vi "test Accessors.vi"(8 "error in (no error)":errorcluster, 11 "TestCase in":refnum<class "Buffers Tests.lvclass">) -> (0 "error out":errorcluster, 3 "TestCase out":refnum<class "Buffers Tests.lvclass">)   [LabVIEW 2017, in "Buffers Tests.lvclass"]
uses:
  Buffers Tests.lvclass
  Buffers Tests.lvclass/Buffers Tests.ctl
  Classes/Buffers/Buffers.lvclass/Buffers.ctl
  Classes/Buffer/Buffer.lvclass
  C:/Git/DSF/LabVIEW-Memory/Source/Classes/Pointer/Pointer.lvclass
  LabVIEW-Memory/Source/Classes/Pointer/Get Address.vi
  LabVIEW-Memory/Source/Classes/Pointer/Get Size.vi
  <vilib>/addons/_JKI Toolkits/VI Tester/TestCase.llb/TestCase.lvclass
  Classes/Buffers/Buffers.lvclass
  C:/Program Files (x86)/National Instruments/LabVIEW 2017/vi.lib/addons/_JKI Toolkits/VI Tester/TestCase.llb/TestCase.lvclass
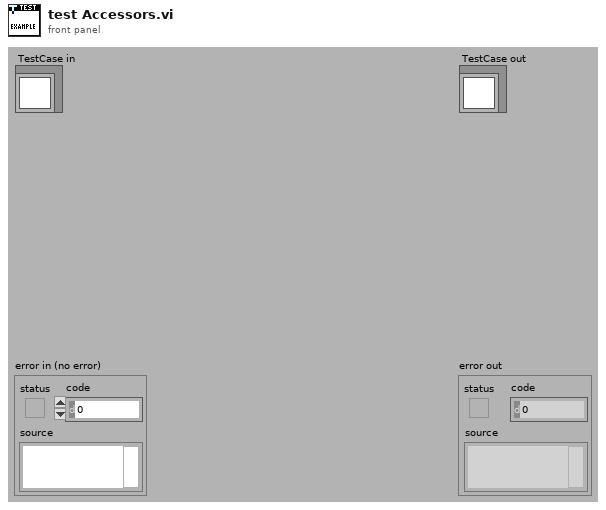
[diagram p1: front panel]
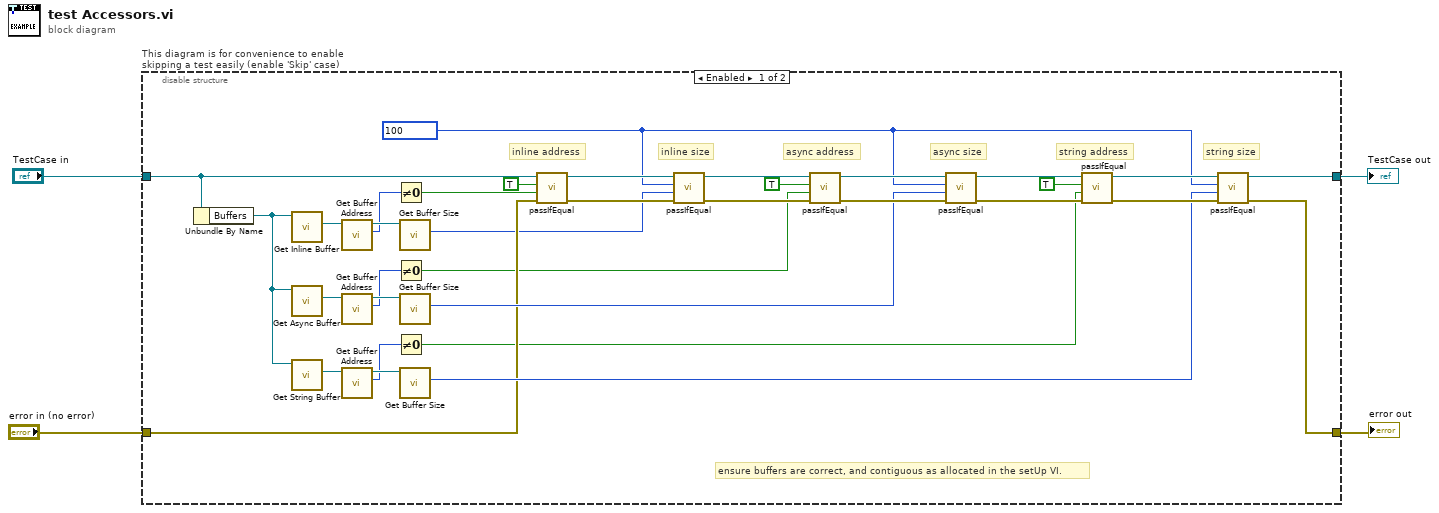
[diagram p0: block diagram]
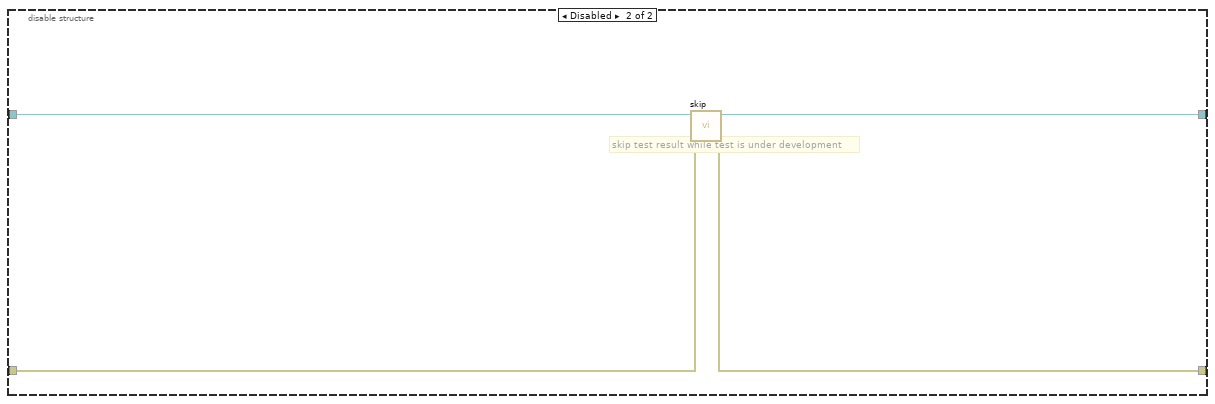
[diagram p2: hidden frame]
diagram:
  n1 = disable-structure "This diagram is for convenience to enable skipping a test easily (enable 'Skip' case)" shown="Enabled" {
    disable-tunnel: "TestCase in" -> [w19 w42]
    disable-tunnel: [w31 w40] -> w1
    disable-tunnel: [w26 w41] -> w3
    disable-tunnel: "error in (no error)" -> [w16 w39]
    frame Enabled {
      w15 = u64 100 ("buffer size")
      # "inline address"
      # "ensure buffers are correct, and contiguous as allocated in the setUp VI."
      # "string size"
      # "string address"
      # "async size"
      # "async address"
      # "inline size"
      n2 = Unbundle By Name(w19) -> ("Buffers"=w37:refnum<class "Buffers.lvclass">)
      n3 = call "Get Inline Buffer.vi"("Buffers in"=w37) -> ("Inline Buffer"=w22:refnum<class "Buffer.lvclass">)  [unwired: 9 in, 1 out]
      n4 = call "Get Async Buffer.vi"("Buffers in"=w37) -> ("Async Buffer"=w21:refnum<class "Buffer.lvclass">)  [unwired: 9 in, 1 out]
      n5 = call "Get String Buffer.vi"("Buffers in"=w37) -> ("String Buffer"=w20:refnum<class "Buffer.lvclass">)  [unwired: 9 in, 1 out]
      n6 = call "Get Buffer Address.vi"("Buffer in"=w22) -> ("buffer address"=w13:u64, "Buffer out"=w38:refnum<class "Buffer.lvclass">)  [unwired: 9 in]
      n7 = call "Get Buffer Address.vi"("Buffer in"=w21) -> ("buffer address"=w11:u64, "Buffer out"=w34:refnum<class "Buffer.lvclass">)  [unwired: 9 in]
      n8 = call "Get Buffer Address.vi"("Buffer in"=w20) -> ("buffer address"=w10:u64, "Buffer out"=w25:refnum<class "Buffer.lvclass">)  [unwired: 9 in]
      n9 = Not Equal To 0?(x=w13) -> (x != 0?=w12:bool)
      n10 = Not Equal To 0?(x=w11) -> (x != 0?=w9:bool)
      n11 = Not Equal To 0?(x=w10) -> (x != 0?=w8:bool)
      n12 = call "Get Buffer Size.vi"("Buffer in"=w38) -> ("buffer size"=w14:u64)  [unwired: 9 in, 1 out]
      n13 = call "Get Buffer Size.vi"("Buffer in"=w34) -> ("buffer size"=w24:u64)  [unwired: 9 in, 1 out]
      n14 = call "Get Buffer Size.vi"("Buffer in"=w25) -> ("buffer size"=w23:u64)  [unwired: 9 in, 1 out]
      n15 = call-dynamic "passIfEqual.vi"("error in (no error)"=w16, "y"=w12, "x"=TRUE, "TestCase in"=w19) -> ("error out"=w17:errorcluster, "TestCase out"=w18:refnum<class "Buffers Tests.lvclass">)  [unwired: 6 in]
      n16 = call-dynamic "passIfEqual.vi"("error in (no error)"=w17, "y"=w14, "x"=w15, "TestCase in"=w18) -> ("error out"=w30:errorcluster, "TestCase out"=w36:refnum<class "Buffers Tests.lvclass">)  [unwired: 6 in]
      n17 = call-dynamic "passIfEqual.vi"("error in (no error)"=w30, "y"=w9, "x"=TRUE, "TestCase in"=w36) -> ("error out"=w29:errorcluster, "TestCase out"=w35:refnum<class "Buffers Tests.lvclass">)  [unwired: 6 in]
      n18 = call-dynamic "passIfEqual.vi"("error in (no error)"=w29, "y"=w24, "x"=w15, "TestCase in"=w35) -> ("error out"=w28:errorcluster, "TestCase out"=w33:refnum<class "Buffers Tests.lvclass">)  [unwired: 6 in]
      n19 = call-dynamic "passIfEqual.vi"("error in (no error)"=w28, "y"=w8, "x"=TRUE, "TestCase in"=w33) -> ("error out"=w27:errorcluster, "TestCase out"=w32:refnum<class "Buffers Tests.lvclass">)  [unwired: 6 in]
      n20 = call-dynamic "passIfEqual.vi"("error in (no error)"=w27, "y"=w23, "x"=w15, "TestCase in"=w32) -> ("error out"=w26:errorcluster, "TestCase out"=w31:refnum<class "Buffers Tests.lvclass">)  [unwired: 6 in]
    }
    frame Disabled {
      # "skip test result while test is under development"
      n21 = call <vilib>:"skip.vi"("error in (no error)"=w39, "TestCase in"=w42) -> ("error out"=w41:errorcluster, "TestCase out"=w40:refnum<class "Buffers Tests.lvclass">)  [unwired: 8 in]
    }
  }
  "error out" <- w3
  "TestCase out" <- w1
